vi "BioMap_BinaryFormat.vi"(11 "Binary file path":path) -> ()   [LabVIEW 2014]
uses:
  ControlDef/ProcessingMode.ctl
  Files/Signal_Segment.ctl
  Files/BinaryHeader_v31.ctl
  _BinaryFileViewer/BinaryRead_State.ctl
  _BinaryFileViewer/ReaderUpperLevelRefs.ctl
  _BinaryFileViewer/BinaryReader_Params.ctl
  preProc_State.ctl
  ControlDef/SampleRateSelector.ctl
  Files/BinaryHeader.ctl
  Apps/Apps_static/ScanParams_SingleLine.ctl
  Apps/ImagingMS/Imaging_Params.ctl
  ProcessMethods/SignalAverager/ProcessStates.ctl
  ControlDef/Signal.ctl
  ControlDef/LaserCtrl_Method.ctl
  ControlDef/States-AToF.ctl
  <instrlib>/ESP300/Public/Data/ESP300_State.ctl
  <instrlib>/ESP300/ESP300.lvlib
  <instrlib>/DG535/Command/DG535_States.ctl
  <instrlib>/DG535/SRS_DG535_Lib.lvlib
  Hardware/BNC(QuantumComposers)/BNC_States.ctl
  Hardware/FemtoLaser(Legacy)/Laser_Status.ctl
  Hardware/DAQmx(Legacy)/DAQmx_Status.ctl
  Files/WriterState.ctl
  Hardware/EPM2000(Legacy)/EPM2K_Status.ctl
  ControlDef/QueueRefs.ctl
  <vilib>/ptbypt/NI_PtbyPt.lvlib
  <instrlib>/GenericDAQ/VI/GenericDAQ_Signal.ctl
  <instrlib>/GenericDAQ/GenericDAQ.lvlib
  <instrlib>/GenericDAQ/VI/GenericDAQ_State.ctl
  <instrlib>/GenericDAQ/VI/GenericDAQ_Ctrl_Queue.ctl
panel:
  in  "Method":enum16{"Imaging (2D)", "Depth Profiling"}(ring)
  out "records/s":dbl format="%0.2f"
  out "CoreState":T1(ring)
  in  "Depth Overide":i32=-1
  in  "Rep.Rate (Hz)":dbl=10.0
  out "record count":i32
  in  "CheckHeader":bool
  in  "File Header":T2={"Start Position"=[], "StepWidth"=[0.05, 0.05], "Dimension"=[], "SpecLength"=10000}
  out "InvalidSpec":i32
  out "Percentage":dbl(slide) scale=0.0..100.0 scale format="%.1f"
  in  "Calibr.":dbl[](array[numeric])
  in  "ForceQuit":bool caption="Quit"
  in  "StartConv.":bool
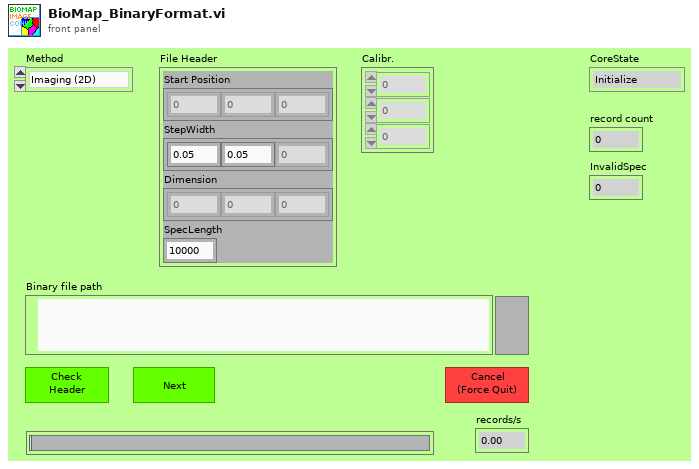
[diagram p1: front panel]
types:
  T1 = enum16{"Initialize", "Open", "Start", "Read", "Close", "Quit"}
  T2 = typedef "BinaryHeader_v31.ctl" = cluster{"Start Position":dbl[], "StepWidth":dbl[], "Dimension":i32[], "SpecLength":i32}
  T3 = typedef "BinaryReader_Params.ctl" = cluster{"FileVersion":string, "Start Position":dbl[], "StepWidth":dbl[], "Dimension":i32[], "TotalDepth":i32, "Spec#":u32, "FileSize":i64, "Calibr.":dbl[], "Position":dbl[], "Pressure":dbl, "Desp_LaserEnergy":dbl, "PI_LaserEnergy":dbl, "SpecLength":dbl, "Average#":i32, "SampleRate":dbl, "DAQ_Range":dbl, "Voltages Table":sgl[][], "ProcMode":T4, "Time Stamp":timestamp, "TrigDelay":dbl, "TickCount":dbl}
  T4 = typedef "ProcessingMode.ctl" = enum16{"None", "Drop by Threshold", "TDC Simulate", "SetFilter"}
  T5 = cluster{"PIEnergyCorrect":bool, "TBD":bool, "SpecLength":i32, "HeaderRefs":refnum<vi>, "Header":T3, "BioMAP file path":path, "InvalidSpec":refnum<vi>, "Calibr.Ref":refnum<vi>, "File Header":refnum<vi>, "QuitUserEvent":refnum<user-event>, "Proc/Signal_CoreQueue":refnum<queue>, "DynamicParams_Queue":refnum<queue>, "WriterQueue":refnum<queue>, "ProcessorHandle":refnum<vi>, "BufferRefs":refnum<queue>}
  T6 = typedef "preProc_State.ctl" = cluster{"State":enum16{"Initialize", "Open", "Start", "Read", "Close", "Quit"}, "Para.":variant}
  T7 = typedef "ReaderUpperLevelRefs.ctl" = cluster{"Percentage":refnum<vi>, "ForceQuit":refnum<vi>, "Header":refnum<vi>}
  T8 = typedef "Signal_Segment.ctl" = cluster{"SampleRate":dbl, "TrigDelay":dbl, "SpecLength":dbl, "DAQ_Range":dbl, "Average#":i32, "Position":dbl[], "Spectrum":sgl[], "Calibr.":dbl[], "Pressure":dbl, "Desp_LaserEnergy":dbl, "PI_LaserEnergy":dbl, "Voltages Table":sgl[][], "ProcMode":T4, "Threshold":dbl, "Comment":string, "TickCount":dbl, "Time Stamp":timestamp}
  T9 = typedef "BinaryRead_State.ctl" = cluster{"State":enum16{"Open", "GetHeader", "Index", "Read_i", "Read_all", "Close", "Quit"}, "Params":variant}
  T10 = cluster{"Image file path":path, "Binary file path":path}
  T11 = typedef "QueueRefs.ctl" = cluster{"LaserCtrlMethod":T12, "Apps":refnum<queue>, "MainDAQCoreQueue":refnum<queue>, "Micos":refnum<queue>, "ESP300":refnum<queue>, "SMC100":refnum<queue>, "SRS DG535":refnum<queue>, "BNC":refnum<queue>, "SDG_ii":refnum<queue>, "NI-USB_DAQmx":refnum<queue>, "ProcCore_CtrlQueue":refnum<queue>, "WriterCtrl":refnum<queue>, "WriterSIG":refnum<queue>, "Feedback":refnum<queue>, "EPM2000":refnum<queue>, "InfoRef":refnum<vi>, "AppsLock":T13, "ProcCore_SignalBuffer":refnum<queue>}
  T12 = typedef "LaserCtrl_Method.ctl" = enum16{"SRS_DG535", "BNC", "SDG_II", "GenericDAQ_Sim"}
  T13 = typedef "Semaphore RefNum" = refnum<k1>
  T14 = typedef "Signal.ctl" = cluster{"Command":T15, "Params":variant}
  T15 = typedef "ProcessStates.ctl" = enum16{"Initialize", "Normal", "Display", "Write2Buffer", "CalcMzArray", "StartSave", "StopSave", "ConfigChanged", "EndOfLine", "SetFilterParams", "SetGraphsEnable", "SetAcquisitionParams", "ChangeDisplayIncrement", "ChangeRepRate", "SetWriterRef", "Quit", "StartOfLine"}
  T16 = typedef "Imaging_Params.ctl" = cluster{"File Header":T17, "ScanSpeed":dbl, "HighSpeed":dbl, "SampleRate":T18, "Rep.Rate (Hz)":dbl, "TrigDelay":dbl, "mzCali":dbl[], "KeepStill(ms)":u32, "SaveRaw":bool, "MultiRec":bool}
  T17 = typedef "BinaryHeader.ctl" = cluster{"Start Position":dbl[], "StepWidth":dbl[], "Dimension":i32[], "SpecLength":i32}
  T18 = typedef "SampleRateSelector.ctl" = dbl
  T19 = typedef "ScanParams_SingleLine.ctl" = cluster{"Line Start":dbl[], "Line End":dbl[], "HighSpeed":dbl, "ScanSpeed":dbl, "KeepStill(ms)":u32, "SecendaryParams":variant}
  T20 = cluster{"queue out":refnum<queue>, "queue out":refnum<queue>}
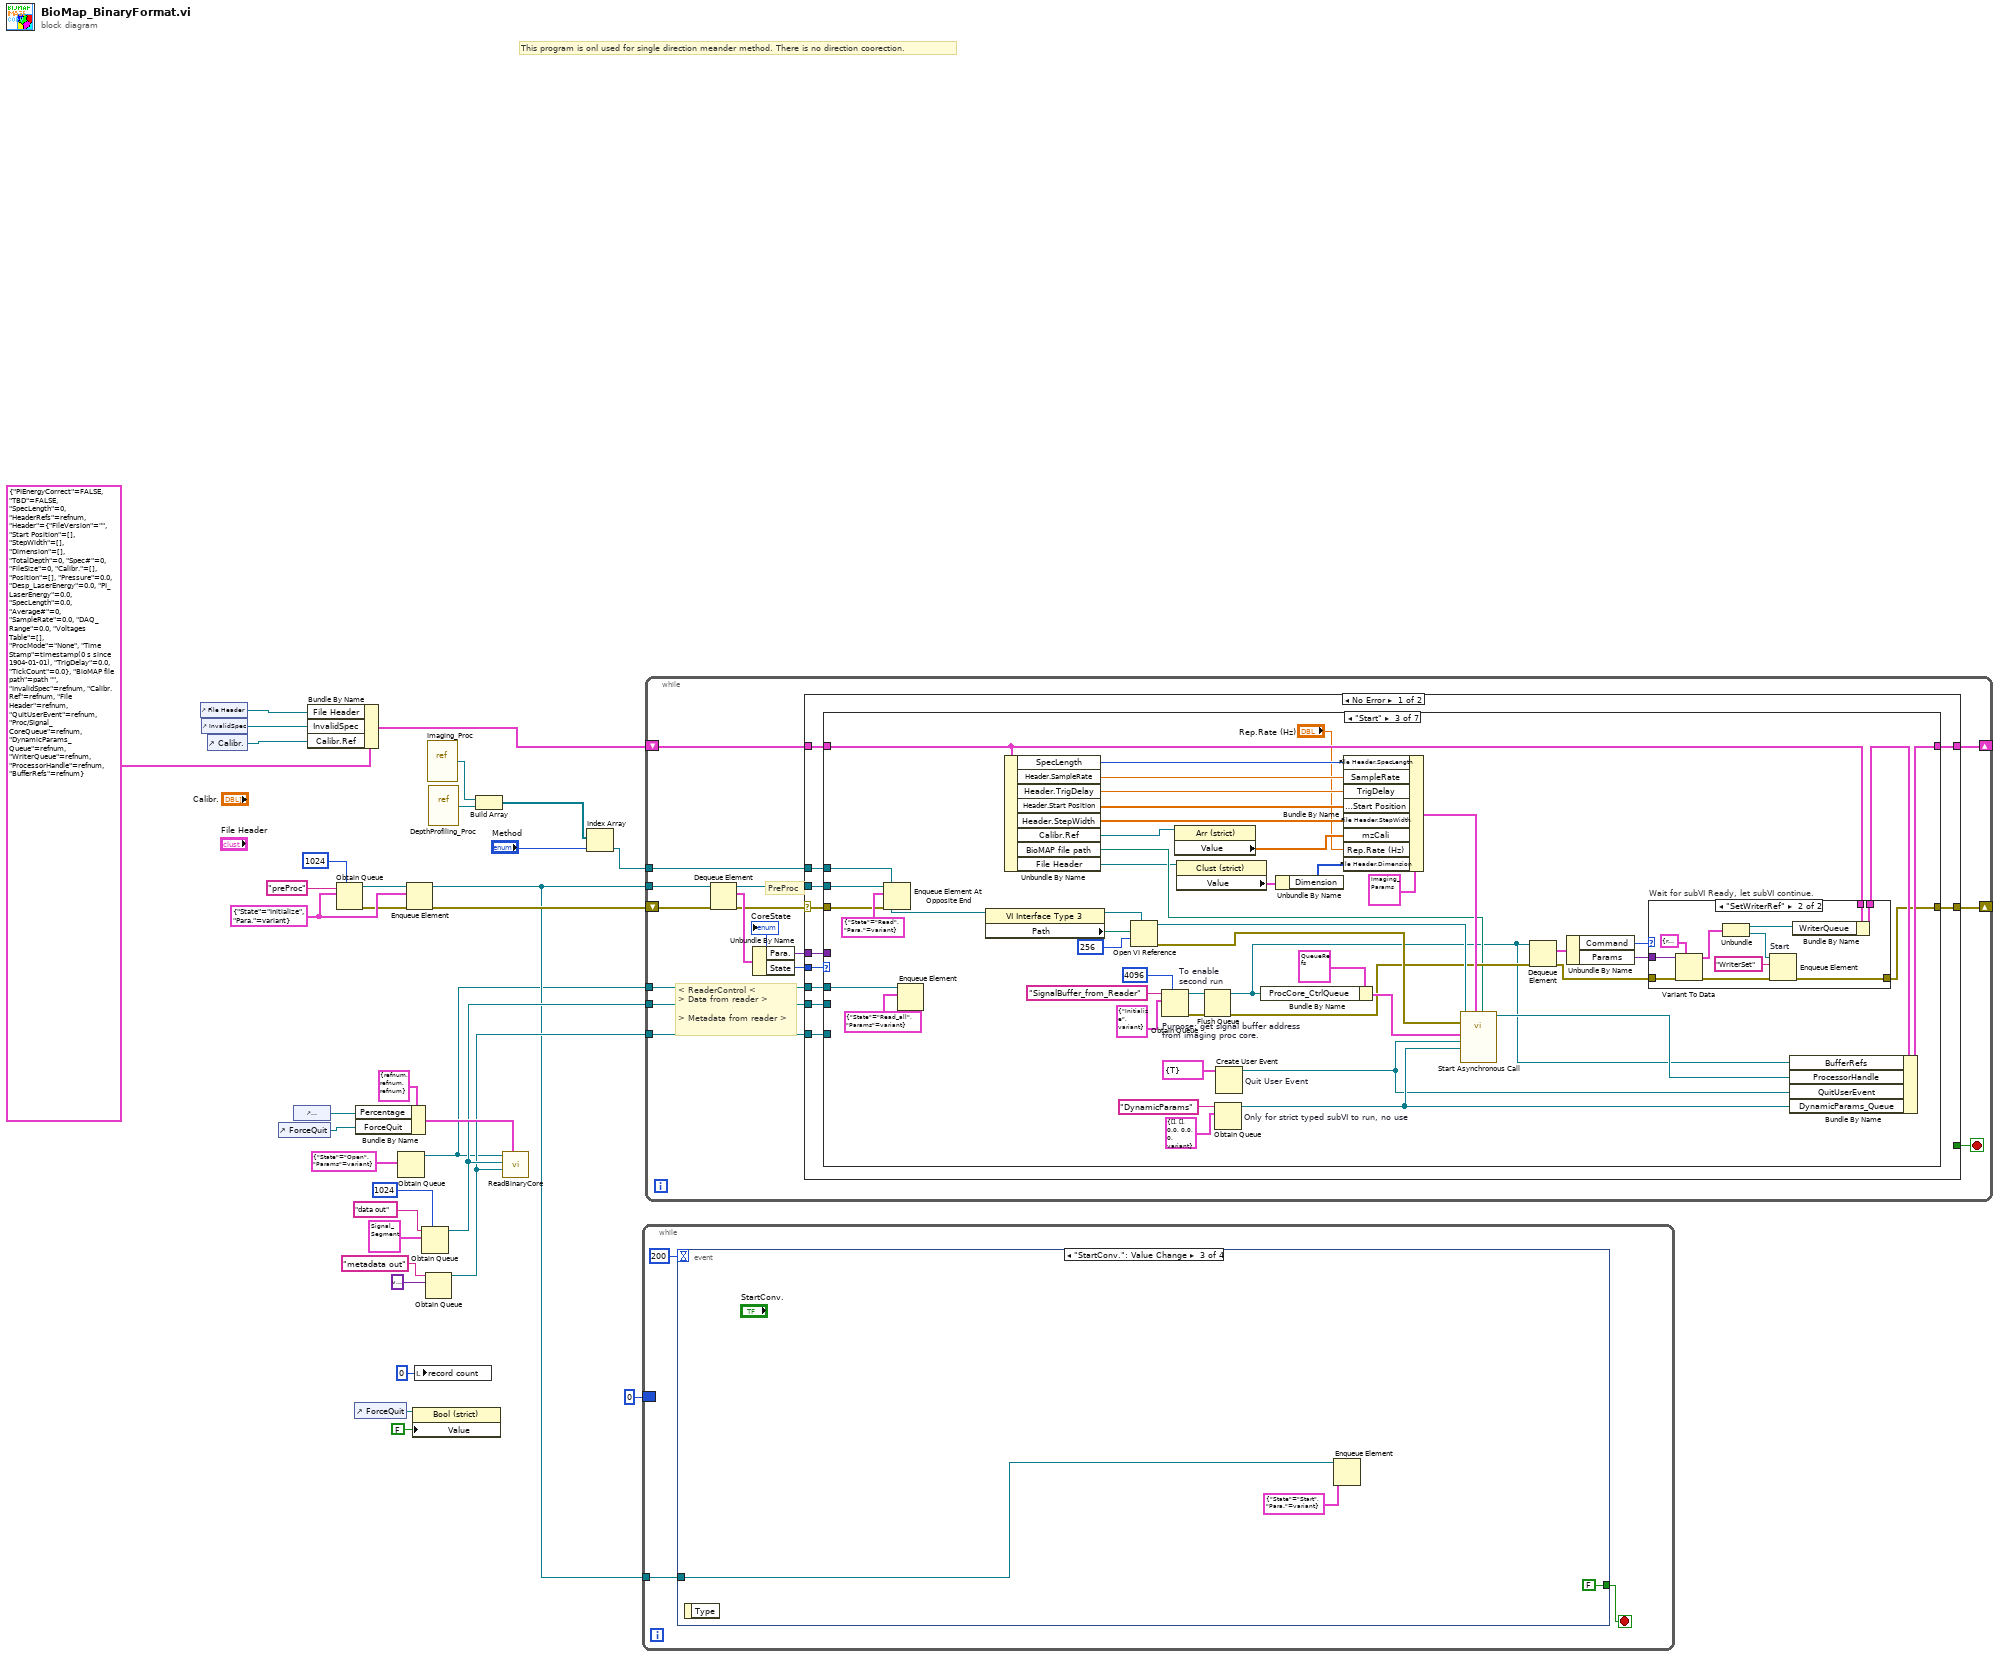
[diagram p0: block diagram]
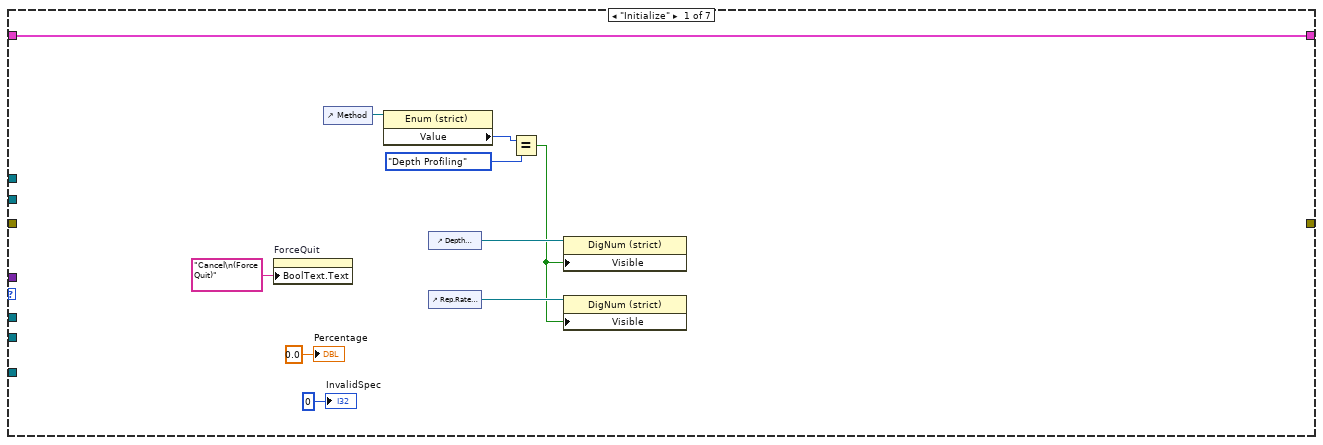
[diagram p2: hidden frame]
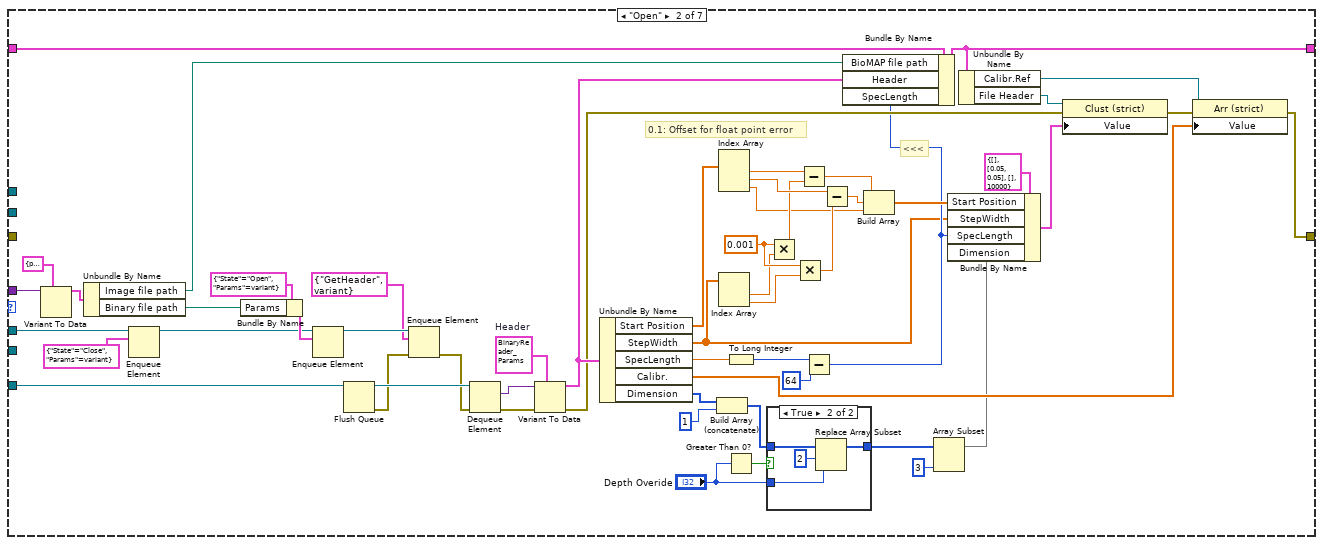
[diagram p3: hidden frame]
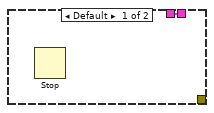
[diagram p5: hidden frame]
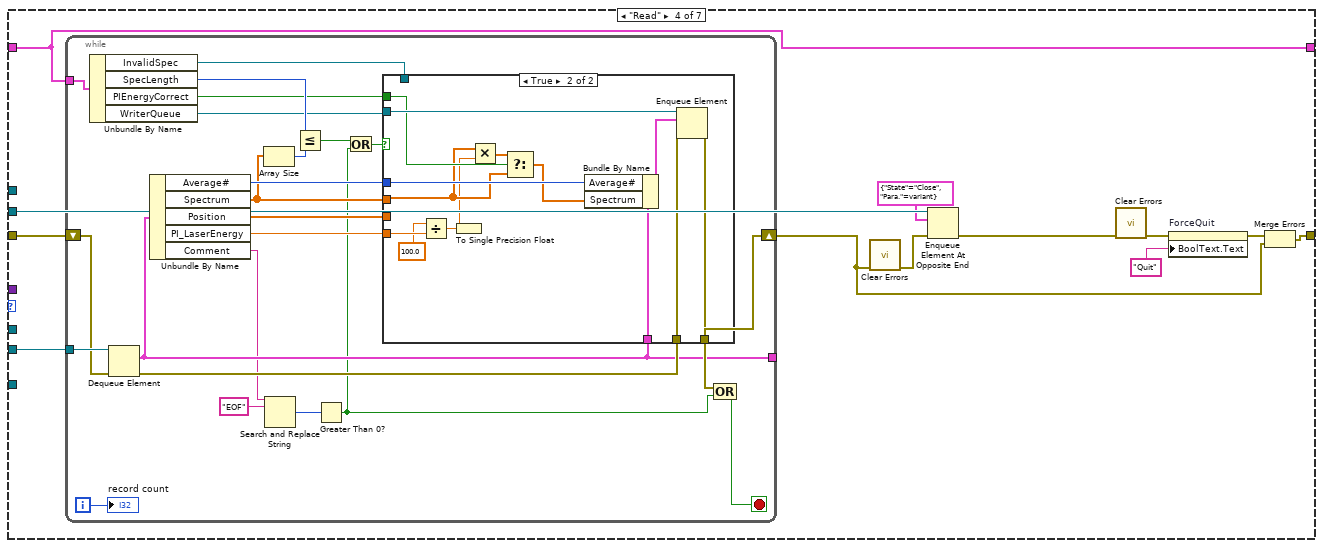
[diagram p6: hidden frame]
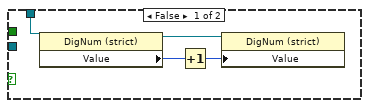
[diagram p7: hidden frame]
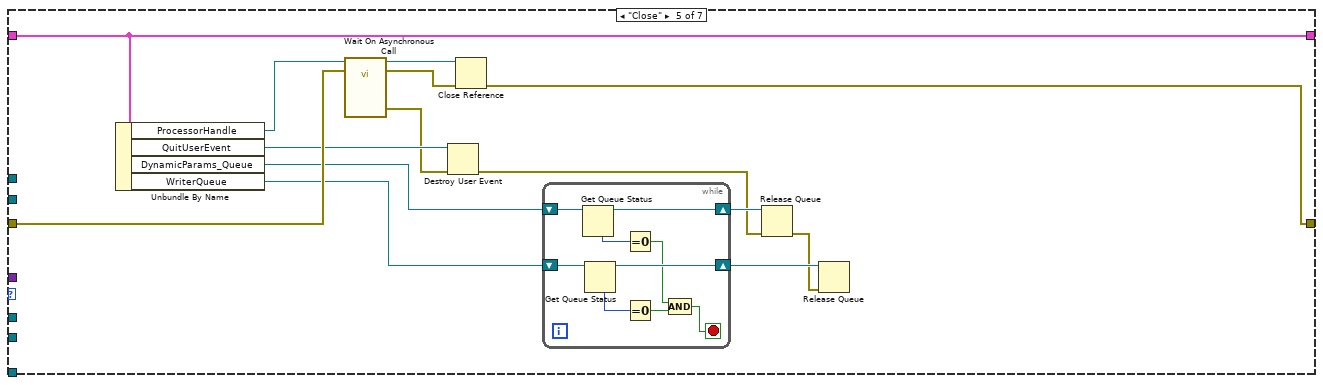
[diagram p8: hidden frame]
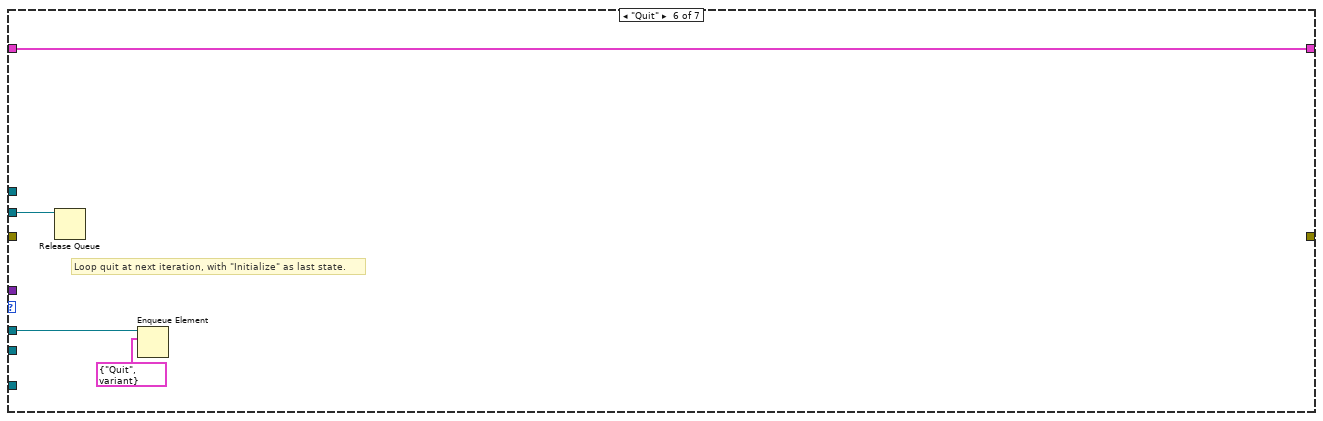
[diagram p9: hidden frame]
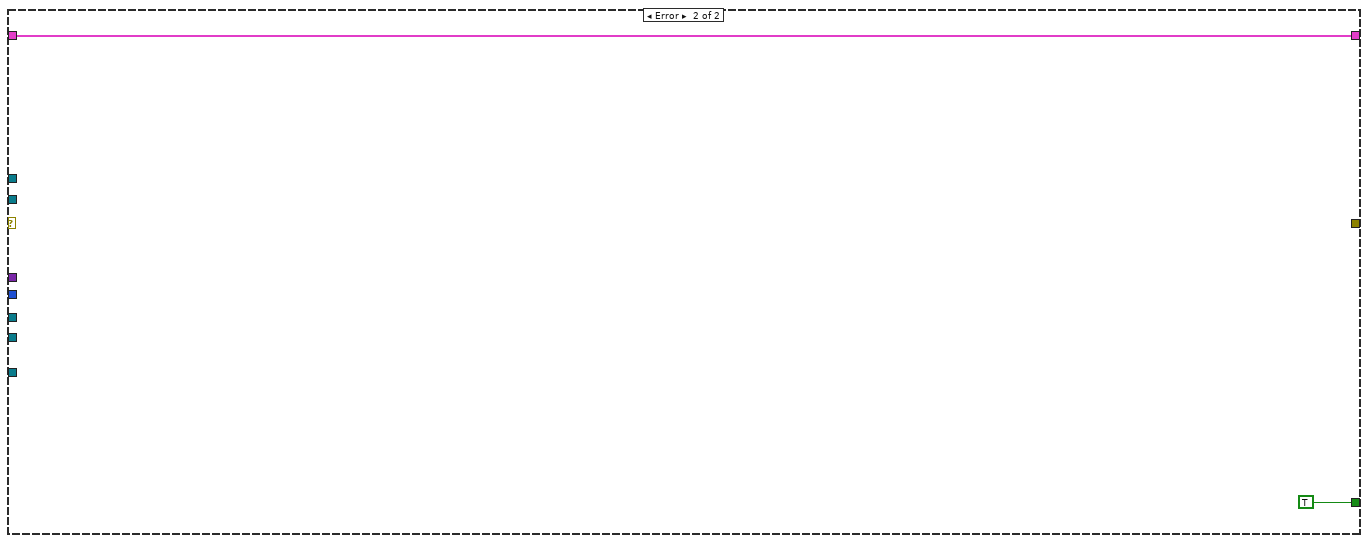
[diagram p11: hidden frame]
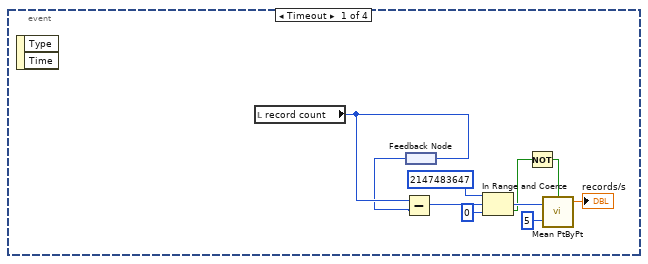
[diagram p12: hidden frame]
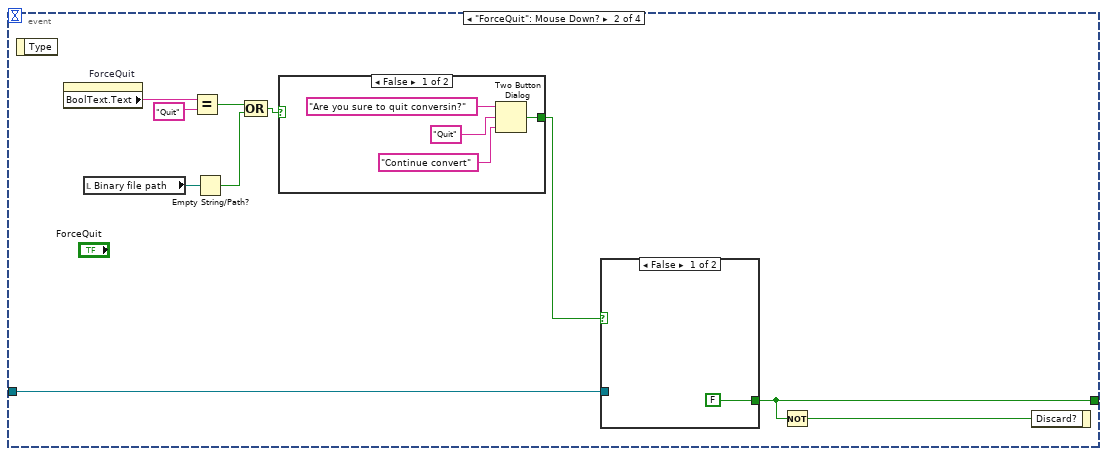
[diagram p13: hidden frame]
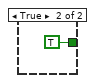
[diagram p14: hidden frame]
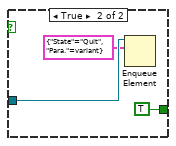
[diagram p15: hidden frame]
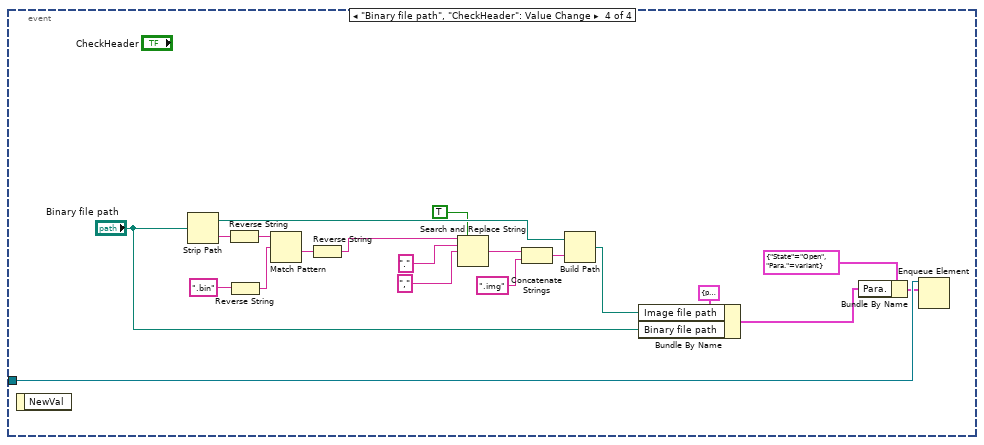
[diagram p16: hidden frame]
diagram:
  w26 = T6 {"State"=enum."Initialize", "Para."=variant}
  # "This program is onl used for single direction meander method. There is no direction coorection."
  n1 = control-ref of="File Header"() -> (w16:refnum<vi>)
  n2 = control-ref of="InvalidSpec"() -> (w19:refnum<vi>)
  n3 = control-ref of="Calibr."() -> (w20:refnum<vi>)
  n4 = control-ref of="ForceQuit"() -> (w14:refnum<vi>)
  n5 = control-ref of="Percentage"() -> (w32:refnum<vi>)
  n6 = Bundle By Name(cluster=T5 {"PIEnergyCorrect"=FALSE, "TBD"=FALSE, "SpecLength"=0, "HeaderRefs"=refnum, "Header"={"FileVersion"="", "Start Position"=[], "StepWidth"=[], "Dimension"=[], "TotalDepth"=0, "Spec#"=0, "FileSize"=0, "Calibr."=[], "Position"=[], "Pressure"=0.0, "Desp_LaserEnergy"=0.0, "PI_LaserEnergy"=0.0, "SpecLength"=0.0, "Average#"=0, "SampleRate"=0.0, "DAQ_Range"=0.0, "Voltages Table"=[], "ProcMode"=enum."None", "Time Stamp"=timestamp(0 s since 1904-01-01), "TrigDelay"=0.0, "TickCount"=0.0}, "BioMAP file path"=path "", "InvalidSpec"=refnum, "Calibr.Ref"=refnum, "File Header"=refnum, "QuitUserEvent"=refnum, "Proc/Signal_CoreQueue"=refnum, "DynamicParams_Queue"=refnum, "WriterQueue"=refnum, "ProcessorHandle"=refnum, "BufferRefs"=refnum}, "File Header"=w16, "InvalidSpec"=w19, "Calibr.Ref"=w20) -> (w17:T5)
  n7 = Obtain Queue(max queue size (-1, unlimited)=1024, name (unnamed)="preProc", element data type=w26) -> (queue out=w24:refnum<queue>, error out=w25:errorcluster)  [unwired: 2 in, 1 out]
  n8 = control-ref of="ForceQuit"() -> (w12:refnum<vi>)
  n9 = Bundle By Name(cluster=T7 {"Percentage"=refnum, "ForceQuit"=refnum, "Header"=refnum}, "Percentage"=w32, "ForceQuit"=w14) -> (w30:T7)
  n10 = Obtain Queue(element data type=T9 {"State"=enum."Open", "Params"=variant}) -> (queue out=w13:refnum<queue>)  [unwired: 4 in, 2 out]
  n11 = Enqueue Element(queue=w24, element=w26, error in (no error)=w25) -> (queue out=w15:refnum<queue>, error out=w23:errorcluster)  [unwired: 1 in, 1 out]
  n12 = property class="Bool (strict)"(reference=w12, "Value"=FALSE) -> ()  [unwired: 1 in, 2 out]
  n13 = local write "record count"(0 ("record count")) -> ()
  n14 = Obtain Queue(max queue size (-1, unlimited)=1024, name (unnamed)="data out", element data type=T8 {"SampleRate"=0.0, "TrigDelay"=0.0, "SpecLength"=0.0, "DAQ_Range"=0.0, "Average#"=0, "Position"=[], "Spectrum"=[], "Calibr."=[], "Pressure"=0.0, "Desp_LaserEnergy"=0.0, "PI_LaserEnergy"=0.0, "Voltages Table"=[], "ProcMode"=enum."None", "Threshold"=0.0, "Comment"="", "TickCount"=0.0, "Time Stamp"=timestamp(0 s since 1904-01-01)} ("Signal Segment")) -> (queue out=w29:refnum<queue>)  [unwired: 2 in, 2 out]
  n15 = Obtain Queue(name (unnamed)="metadata out", element data type=variant) -> (queue out=w21:refnum<queue>)  [unwired: 3 in, 2 out]
  n16 = vi-ref "Imaging_Proc.vi"() -> (w5:refnum<vi>)
  n17 = vi-ref "DepthProfiling_Proc.vi"() -> (w4:refnum<vi>)
  n18 = Build Array(w5, w4) -> (w2:refnum<vi>[])
  n19 = call "ReadBinaryCore.vi"("UpperLevelControlRefs."=w30, "metadata in"=w21, "data out in"=w29, "Control Queue in"=w13) -> ()  [unwired: 8 in]
  n20 = Index Array(array=w2, index="Method") -> (element=w3:refnum<vi>)
  n21 = while {
    tunnel: w15 -> [w36]
    border: 0 ("record count") -> [_]
    stop <- w37 stop-if-true
    n22 = event shown="[2] \"StartConv.\": Value Change" {
      selector: _ -> [_ _ _ _]
      dyn-events: _ -> [_ _ _ _]
      timeout: 200 -> [_ _ _ _]
      tunnel: [_ w57 FALSE _] -> w37
      tunnel: w36 -> [_ w48 w69 w81]
      event Timeout {
        n23 = event-data() -> ()  [unwired: 1 in, 2 out]
        n24 = local read "record count"() -> (w44:i32)
        n25 = feedback-in #1(w44) -> ()
        n26 = feedback #1() -> (w43:i32)
        n27 = Subtract(x=w44, y=w43) -> (x-y=w47:i32)
        n28 = In Range and Coerce(upper limit=2147483647, x=w47, lower limit=0) -> (coerced(x)=w42:i32, In Range?=w39:bool)
        n29 = Not(x=w39) -> (.not. x?=w38:bool)
        n30 = call <vilib>:"Mean PtByPt.vi"("x"=w42, "sample length"=5, "initialize"=w38) -> ("mean"=→"records/s":dbl)  [unwired: 1 in, 1 out]
      }
      event "ForceQuit": Mouse Down? {
        n31 = event-data() -> ()  [unwired: 1 in, 1 out]
        n32 = property on="ForceQuit" class="Bool (strict)"() -> ("BoolText.Text"=w53:string)  [unwired: 2 in, 2 out]
        n33 = local read "Binary file path"() -> (w52:path)
        n34 = Equal?(x=w53, y="Quit" ("Caption.Text")) -> (x = y?=w50:bool)
        n35 = Empty String/Path?(string/path=w52) -> (empty?=w49:bool)
        n36 = Compound Arithmetic op=OR(w50, w49) -> (w51:bool)
        n37 = case shown="False" w51 {
          tunnel: [w58 TRUE ("T button?")] -> w55
          frame False {
            n38 = Two Button Dialog(message="Are you sure to quit conversin?", 1:"Continue convert" ("F button name (\"Cancel\")"), 2:"Quit" ("T button name (\"OK\")")) -> (T button?=w58:bool)
          }
          frame True {
          }
        }
        n39 = case shown="False" w55 {
          tunnel: [FALSE TRUE] -> w57
          tunnel: w48 -> [_ w65]
          frame False {
          }
          frame True {
            n40 = Enqueue Element(queue=w65, element=T6 {"State"=enum."Quit", "Para."=variant}) -> ()  [unwired: 2 in, 3 out]
          }
        }
        n41 = Not(x=w57) -> (.not. x?=w56:bool)
        n42 = event-data("Discard?"=w56) -> ()  [unwired: 1 in, 1 out]
      }
      event "StartConv.": Value Change {
        n43 = event-data() -> ()  [unwired: 1 in, 1 out]
        n44 = Enqueue Element(queue=w69, element=T6 {"State"=enum."Start", "Para."=variant}) -> ()  [unwired: 2 in, 3 out]
      }
      event "Binary file path", "CheckHeader": Value Change {
        n45 = event-data() -> ()  [unwired: 1 in, 1 out]
        n46 = Strip Path(path="Binary file path") -> (stripped path=w82:path, name=w83:string)
        n47 = Reverse String(1:w83) -> (0:w89:string)
        n48 = Reverse String(1:".bin" ("regular expression")) -> (0:w84:string)
        n49 = Match Pattern(string=w89, regular expression=w84) -> (after substring=w86:string)  [unwired: 1 in, 3 out]
        n50 = Reverse String(1:w86) -> (0:w73:string)
        n51 = Search and Replace String(replace all?=TRUE ("replace all? (F)"), input string=w73, search string=".", replace string="," ("replace string (\"\")")) -> (result string=w74:string)  [unwired: 4 in, 3 out]
        n52 = Concatenate Strings(w74, ".img" ("string")) -> (w87:string)
        n53 = Build Path(base path=w82, name or relative path=w87) -> (appended path=w78:path)
        n54 = Bundle By Name(cluster=T10 {"Image file path"=path "", "Binary file path"=path ""} ("input cluster"), "Image file path"=w78, "Binary file path"="Binary file path") -> (w75:T10)
        n55 = Bundle By Name(cluster=T6 {"State"=enum."Open", "Para."=variant} ("element"), "Para."=w75) -> (w79:T6)
        n56 = Enqueue Element(queue=w81, element=w79) -> ()  [unwired: 2 in, 3 out]
      }
    }
  }
  n57 = while {
    tunnel: w29 -> [w104]
    tunnel: w15 -> [w102]
    shift-right: [w91] -> _
    shift-left: w23 -> [w103]
    tunnel: w13 -> [w98]
    shift-right: [w96] -> _
    shift-left: w17 -> [w95]
    tunnel: w21 -> [w94]
    tunnel: w3 -> [w90]
    stop <- w92 stop-if-true
    # "< ReaderControl <\n> Data from reader >\n\n> Metadata from reader >"
    # "PreProc"
    n58 = Dequeue Element(queue=w102, error in (no error)=w103) -> (queue out=w97:refnum<queue>, element=w101:T6, error out=w93:errorcluster)  [unwired: 1 in, 1 out]
    n59 = Unbundle By Name(w101) -> ("Para."=w99:variant, "State"=w100:T1)
    "CoreState" <- w100
    n60 = case shown="No Error" w93 {
      selector: w93 -> [w107 _]
      tunnel: w104 -> [w115 _]
      tunnel: w100 -> [w114 _]
      tunnel: w99 -> [w113 _]
      tunnel: w98 -> [w112 _]
      tunnel: w97 -> [w111 _]
      tunnel: [w110 w327] -> w96
      tunnel: w95 -> [w109 w327]
      tunnel: w94 -> [w108 _]
      tunnel: [_ TRUE] -> w92
      tunnel: [w106 _] -> w91
      tunnel: w90 -> [w105 _]
      frame No Error {
        n61 = case shown="\"Start\"" w114 {
          tunnel: w115 -> [_ _ _ w257 _ _ _]
          tunnel: w107 -> [_ _ w230 w256 w310 _ _]
          tunnel: w113 -> [_ w180 _ _ _ _ _]
          tunnel: w112 -> [_ w179 w204 _ _ w324 _]
          tunnel: w111 -> [_ _ w231 w255 _ w325 _]
          tunnel: [w122 w165 w212 w248 w312 w322 w326] -> w110
          tunnel: w109 -> [w122 w168 w209 w248 w312 w322 w326]
          tunnel: w108 -> [_ w175 _ _ _ _ _]
          tunnel: [_ w142 w199 w250 w307 _ _] -> w106
          tunnel: w105 -> [_ _ w192 _ _ _ _]
          frame "Initialize" {
            n62 = property on="ForceQuit" class="Bool (strict)"("BoolText.Text"="Cancel\n(Force Quit)" ("Caption.Text")) -> ()  [unwired: 2 in, 2 out]
            n63 = control-ref of="Method"() -> (w119:refnum<vi>)
            n64 = property class="Enum (strict)"(reference=w119) -> ("Value"=w118:enum16{"Imaging (2D)", "Depth Profiling"})  [unwired: 1 in, 2 out]
            n65 = control-ref of="Depth Overide"() -> (w121:refnum<vi>)
            n66 = control-ref of="Rep.Rate (Hz)"() -> (w120:refnum<vi>)
            n67 = Equal?(x=w118, y=enum16{"Imaging (2D)", "Depth Profiling"}."Depth Profiling") -> (x = y?=w116:bool)
            n68 = property class="DigNum (strict)"(reference=w121, "Visible"=w116) -> ()  [unwired: 1 in, 2 out]
            n69 = property class="DigNum (strict)"(reference=w120, "Visible"=w116) -> ()  [unwired: 1 in, 2 out]
            "Percentage" <- 0.0 ("Percentage")
            "InvalidSpec" <- 0 ("InvalidSpec")
          }
          frame "Open" {
            w161 = 0.001 ("x")
            w170 = T3 {"FileVersion"="", "Start Position"=[], "StepWidth"=[], "Dimension"=[], "TotalDepth"=0, "Spec#"=0, "FileSize"=0, "Calibr."=[], "Position"=[], "Pressure"=0.0, "Desp_LaserEnergy"=0.0, "PI_LaserEnergy"=0.0, "SpecLength"=0.0, "Average#"=0, "SampleRate"=0.0, "DAQ_Range"=0.0, "Voltages Table"=[], "ProcMode"=enum."None", "Time Stamp"=timestamp(0 s since 1904-01-01), "TrigDelay"=0.0, "TickCount"=0.0}  # Header
            # "<<<"
            # "0.1: Offset for float point error"
            n70 = Variant To Data(type=T10 {"Image file path"=path "", "Binary file path"=path ""} ("input cluster"), Variant=w180) -> (data=w139:T10)  [unwired: 1 in, 1 out]
            n71 = Unbundle By Name(w139) -> ("Image file path"=w137:path, "Binary file path"=w138:path)
            n72 = Enqueue Element(queue=w179, element=T9 {"State"=enum."Close", "Params"=variant}) -> (queue out=w167:refnum<queue>)  [unwired: 2 in, 2 out]
            n73 = Bundle By Name(cluster=T9 {"State"=enum."Open", "Params"=variant} ("element"), "Params"=w138) -> (w177:T9)
            n74 = Enqueue Element(queue=w167, element=w177) -> (queue out=w176:refnum<queue>)  [unwired: 2 in, 2 out]
            n75 = Flush Queue(queue=w175) -> (queue out=w174:refnum<queue>, error out=w173:errorcluster)  [unwired: 1 in, 1 out]
            n76 = Enqueue Element(queue=w176, element=T9 {"State"=enum."GetHeader", "Params"=variant}, error in (no error)=w173) -> (error out=w172:errorcluster)  [unwired: 1 in, 2 out]
            n77 = Dequeue Element(queue=w174, error in (no error)=w172) -> (element=w171:variant, error out=w169:errorcluster)  [unwired: 1 in, 2 out]
            n78 = Variant To Data(error in=w169, type=w170, Variant=w171) -> (data=w150:T3, error out=w141:errorcluster)
            n79 = Unbundle By Name(w150) -> ("Start Position"=w155:dbl[], "StepWidth"=w134:dbl[], "SpecLength"=w152:dbl, "Calibr."=w144:dbl[], "Dimension"=w133:i32[])
            n80 = Build Array (concatenate)(w133, 1) -> (w129:i32[])
            n81 = Index Array(array=w155) -> (element #1=w154:dbl, element #2=w162:dbl, element #3=w135:dbl)  [unwired: 3 in]
            n82 = Index Array(array=w134) -> (element #1=w160:dbl, element #2=w163:dbl)  [unwired: 2 in]
            n83 = To Long Integer(number=w152) -> (32bit integer=w151:i32)
            n84 = Greater Than 0?(x="Depth Overide") -> (x > 0?=w130:bool)
            n85 = case shown="True" w130 {
              tunnel: w129 -> [w181 w185]
              tunnel: [w181 w184] -> w132
              tunnel: "Depth Overide" -> [_ w182]
              frame False {
              }
              frame True {
                n86 = Replace Array Subset(array=w185, new element=w182, index=2) -> (w184:i32[])
              }
            }
            n87 = Multiply(x=w161, y=w160) -> (x*y=w158:dbl)
            n88 = Multiply(x=w161, y=w163) -> (x*y=w159:dbl)
            n89 = Subtract(x=w154, y=w158) -> (x-y=w156:dbl)
            n90 = Subtract(x=w151, y=64 ("x")) -> (x-y=w136:i32)
            n91 = Subtract(x=w162, y=w159) -> (x-y=w157:dbl)
            n92 = Bundle By Name(cluster=w168, "BioMAP file path"=w137, "Header"=w150, "SpecLength"=w136) -> (w165:T5)
            n93 = Build Array(w156, w157, w135) -> (w149:dbl[])
            n94 = Array Subset(array=w132, length=3) -> (w127:i32[])  [unwired: 1 in]
            n95 = Bundle By Name(cluster=T2 {"Start Position"=[], "StepWidth"=[0.05, 0.05], "Dimension"=[], "SpecLength"=10000} ("File Header"), "Start Position"=w149, "StepWidth"=w134, "SpecLength"=w136, "Dimension"=w127) -> (w148:T2)
            n96 = Unbundle By Name(w165) -> ("Calibr.Ref"=w145:refnum<vi>, "File Header"=w164:refnum<vi>)
            n97 = property class="Clust (strict)"(reference=w164, error in=w141, "Value"=w148) -> (error out=w146:errorcluster)  [unwired: 1 out]
            n98 = property class="Arr (strict)"(reference=w145, error in=w146, "Value"=w144) -> (error out=w142:errorcluster)  [unwired: 1 out]
          }
          frame "Start" {
            n99 = Enqueue Element At Opposite End(queue=w231, element=T6 {"State"=enum."Read", "Para."=variant}, error in (no error)=w230) -> ()  [unwired: 1 in, 3 out]
            n100 = Enqueue Element(queue=w204, element=T9 {"State"=enum."Read_all", "Params"=variant}) -> ()  [unwired: 2 in, 3 out]
            n101 = property class="VI Interface Type 3"(reference=w192) -> (reference out=w191:refnum<vi>, "Path"=w202:path)  [unwired: 1 in, 1 out]
            n102 = Unbundle By Name(w209) -> ("SpecLength"=w217:i32, "Header.SampleRate"=w218:dbl, "Header.TrigDelay"=w219:dbl, "Header.Start Position"=w221:dbl[], "Header.StepWidth"=w220:dbl[], "Calibr.Ref"=w216:refnum<vi>, "BioMAP file path"=w190:path, "File Header"=w189:refnum<vi>)
            n103 = Open VI Reference(type specifier VI Refnum (for type only)=w191, vi path=w202, options=256) -> (vi reference=w201:refnum<vi>, error out=w200:errorcluster)  [unwired: 3 in]
            n104 = Obtain Queue "Purpose: get signal buffer address \nfrom imaging proc core."(max queue size (-1, unlimited)=4096, name (unnamed)="SignalBuffer_from_Reader", element data type=T14 {"Command"=enum."Initialize", "Params"=variant} ("m/z signal")) -> (queue out=w214:refnum<queue>, error out=w195:errorcluster)  [unwired: 2 in, 1 out]
            n105 = property class="Arr (strict)"(reference=w216) -> ("Value"=w215:dbl[])  [unwired: 1 in, 2 out]
            n106 = property on="Property Node" class="Clust (strict)"(reference=w189) -> ("Value"=w188:T2)  [unwired: 1 in, 2 out]
            n107 = Flush Queue "To enable\nsecond run"(queue=w214, error in (no error)=w195) -> (queue out=w186:refnum<queue>, error out=w194:errorcluster)  [unwired: 1 out]
            n108 = Obtain Queue "Only for strict typed subVI to run, no use"(name (unnamed)="DynamicParams", element data type=T19 {"Line Start"=[], "Line End"=[], "HighSpeed"=0.0, "ScanSpeed"=0.0, "KeepStill(ms)"=0, "SecendaryParams"=variant(dbl[] [])}) -> (queue out=w207:refnum<queue>)  [unwired: 3 in, 2 out]
            n109 = Create User Event "Quit User Event"(user event datatype=cluster{"Quit":bool} {"Quit"=TRUE} ("Quit")) -> (user event=w205:refnum<user-event>)  [unwired: 1 in, 1 out]
            n110 = Bundle By Name(cluster=T11 {"LaserCtrlMethod"=enum."SRS_DG535", "Apps"=refnum, "MainDAQCoreQueue"=refnum, "Micos"=refnum, "ESP300"=refnum, "SMC100"=refnum, "SRS DG535"=refnum, "BNC"=refnum, "SDG_ii"=refnum, "NI-USB_DAQmx"=refnum, "ProcCore_CtrlQueue"=refnum, "WriterCtrl"=refnum, "WriterSIG"=refnum, "Feedback"=refnum, "EPM2000"=refnum, "InfoRef"=refnum, "AppsLock"=refnum, "ProcCore_SignalBuffer"=refnum} ("QueuesRef"), "ProcCore_CtrlQueue"=w186) -> (w198:T11)
            n111 = Unbundle By Name(w188) -> ("Dimension"=w187:i32[])
            n112 = Bundle By Name(cluster=T16 {"File Header"={"Start Position"=[], "StepWidth"=[], "Dimension"=[], "SpecLength"=0}, "ScanSpeed"=0.0, "HighSpeed"=0.0, "SampleRate"=0.0, "Rep.Rate (Hz)"=0.0, "TrigDelay"=0.0, "mzCali"=[], "KeepStill(ms)"=0, "SaveRaw"=FALSE, "MultiRec"=FALSE} ("BeamProfiling_Params"), "File Header.SpecLength"=w217, "SampleRate"=w218, "TrigDelay"=w219, "File Header.Start Position"=w221, "File Header.StepWidth"=w220, "mzCali"=w215, "Rep.Rate (Hz)"="Rep.Rate (Hz)", "File Header.Dimension"=w187) -> (w229:T16)
            n113 = call-by-ref "Start Asynchronous Call"(reference=w201, error in=w200, "DP_filepath"=w190, "Params."=w229, "Dynamic Params In"=w207, "Quit_UserEvent"=w205, "ControlQueueRef"=w198) -> (reference out=w196:refnum<vi>)  [unwired: 5 in, 3 out]
            n114 = Dequeue Element(queue=w186, error in (no error)=w194) -> (element=w213:T14, error out=w193:errorcluster)  [unwired: 1 in, 2 out]
            n115 = Unbundle By Name(w213) -> ("Command"=w211:T15, "Params"=w210:variant)
            n116 = case "Wait for subVI Ready, let subVI continue." shown="\"SetWriterRef\"" w211 {
              tunnel: w209 -> [w234 w245]
              tunnel: w210 -> [_ w244]
              tunnel: [w234 w243] -> w208
              tunnel: [_ w237] -> w199
              tunnel: w193 -> [_ w235]
              frame Default {
                n117 = Stop() -> ()  [unwired: 1 in]
              }
              frame "SetWriterRef" {
                n118 = Variant To Data(error in=w235, type=T20 {"queue out"=refnum, "queue out"=refnum} ("cluster"), Variant=w244) -> (data=w241:T20, error out=w238:errorcluster)
                n119 = Unbundle(w241) -> ("queue out"=w240:refnum<queue>, "queue out"=w239:refnum<queue>)
                n120 = Enqueue Element "Start"(queue=w239, element="WriterSet", error in (no error)=w238) -> (error out=w237:errorcluster)  [unwired: 1 in, 2 out]
                n121 = Bundle By Name(cluster=w245, "WriterQueue"=w240) -> (w243:T5)
              }
            }
            n122 = Bundle By Name(cluster=w208, "BufferRefs"=w186, "ProcessorHandle"=w196, "QuitUserEvent"=w205, "DynamicParams_Queue"=w207) -> (w212:T5)
          }
          frame "Read" {
            n123 = while {
              tunnel: w257 -> [w280]
              shift-right: [w271] -> w249
              shift-left: w256 -> [w276]
              tunnel: w248 -> [w270]
              tunnel: [w263] -> _
              i -> [w264]
              stop <- w272 stop-if-true
              n124 = Unbundle By Name(w270) -> ("InvalidSpec"=w267:refnum<vi>, "SpecLength"=w269:i32, "PIEnergyCorrect"=w268:bool, "WriterQueue"=w266:refnum<queue>)
              n125 = Dequeue Element(queue=w280, error in (no error)=w276) -> (element=w263:T8, error out=w277:errorcluster)  [unwired: 1 in, 2 out]
              n126 = Unbundle By Name(w263) -> ("Average#"=w279:i32, "Spectrum"=w278:sgl[], "Position"=w265:dbl[], "PI_LaserEnergy"=w273:dbl, "Comment"=w262:string)
              n127 = Array Size(array=w278) -> (size(s)=w275:i32)
              n128 = Search and Replace String(input string=w262, search string="EOF" ("y")) -> (number of replacements=w260:i32)  [unwired: 6 in, 3 out]
              n129 = Less Or Equal?(x=w269, y=w275) -> (x <= y?=w274:bool)
              n130 = Greater Than 0?(x=w260) -> (x > 0?=w258:bool)
              n131 = Or(x=w274, y=w258) -> (x .or. y?=w259:bool)
              n132 = case shown="True" w259 {
                tunnel: w266 -> [_ w298]
                tunnel: w279 -> [_ w297]
                tunnel: w278 -> [_ w292]
                tunnel: w277 -> [_ w296]
                tunnel: w273 -> [_ w290]
                tunnel: w268 -> [_ w294]
                tunnel: [_ w288] -> w271
                tunnel: w267 -> [w284 _]
                tunnel: w263 -> [_ w286]
                tunnel: w265 -> [_ _]
                frame False {
                  n133 = property class="DigNum (strict)"(reference=w284) -> (reference out=w283:refnum<vi>, "Value"=w282:i32)  [unwired: 1 in, 1 out]
                  n134 = Increment(x=w282) -> (x+1=w281:i32)
                  n135 = property class="DigNum (strict)"(reference=w283, "Value"=w281) -> ()  [unwired: 1 in, 2 out]
                }
                frame True {
                  n136 = Divide(x=100.0, y=w290) -> (x/y=w291:dbl)
                  n137 = To Single Precision Float(number=w291) -> (single precision float=w287:sgl)
                  n138 = Multiply(x=w292, y=w287) -> (x*y=w293:sgl[])
                  n139 = Select(t=w293, s=w294, f=w292) -> (s? t:f=w295:sgl[])
                  n140 = Bundle By Name(cluster=w286, "Average#"=w297, "Spectrum"=w295) -> (w285:T8)
                  n141 = Enqueue Element(queue=w298, element=w285, error in (no error)=w296) -> (error out=w288:errorcluster)  [unwired: 1 in, 2 out]
                }
              }
              n142 = Compound Arithmetic op=OR(w271, w258) -> (w272:bool)
              "record count" <- w264
            }
            n143 = call <vilib>:"Clear Errors.vi"("error in (no error)"=w249) -> ("error out"=w247:errorcluster)  [unwired: 5 in, 1 out]
            n144 = Enqueue Element At Opposite End(queue=w255, element=T6 {"State"=enum."Close", "Para."=variant}, error in (no error)=w247) -> (error out=w246:errorcluster)  [unwired: 1 in, 2 out]
            n145 = call <vilib>:"Clear Errors.vi"("error in (no error)"=w246) -> ("error out"=w252:errorcluster)  [unwired: 5 in, 1 out]
            n146 = property on="ForceQuit" class="Bool (strict)"(error in=w252, "BoolText.Text"="Quit" ("Caption.Text")) -> (error out=w251:errorcluster)  [unwired: 1 in, 1 out]
            n147 = Merge Errors(w251, w249) -> (w250:errorcluster)
          }
          frame "Close" {
            n148 = Unbundle By Name(w312) -> ("ProcessorHandle"=w311:refnum<vi>, "QuitUserEvent"=w306:refnum<user-event>, "DynamicParams_Queue"=w305:refnum<queue>, "WriterQueue"=w303:refnum<queue>)
            n149 = call-by-ref "Wait On Asynchronous Call"(reference=w311, error in=w310) -> (reference out=w309:refnum<vi>, error out=w308:errorcluster, 0:"error out"=w304:errorcluster)  [unwired: 10 in, 1 out]
            n150 = Destroy User Event(user event=w306, error in=w304) -> (error out=w299:errorcluster)
            n151 = Close Reference(reference=w309, error in (no error)=w308) -> (error out=w307:errorcluster)
            n152 = while {
              shift-right: [w319] -> w302
              shift-left: w305 -> [w321]
              shift-right: [w318] -> w301
              shift-left: w303 -> [w320]
              stop <- w313 stop-if-true
              n153 = Get Queue Status(queue=w321) -> (queue out=w319:refnum<queue>, # elements in queue=w316:i32)  [unwired: 2 in, 6 out]
              n154 = Get Queue Status(queue=w320) -> (queue out=w318:refnum<queue>, # elements in queue=w317:i32)  [unwired: 2 in, 6 out]
              n155 = Equal To 0?(x=w316) -> (x = 0?=w314:bool)
              n156 = Equal To 0?(x=w317) -> (x = 0?=w315:bool)
              n157 = Compound Arithmetic op=AND(w314, w315) -> (w313:bool)
            }
            n158 = Release Queue(queue=w302, error in (no error)=w299) -> (error out=w300:errorcluster)  [unwired: 1 in, 2 out]
            n159 = Release Queue(queue=w301, error in (no error)=w300) -> ()  [unwired: 1 in, 3 out]
          }
          frame "Quit" {
            # "Loop quit at next iteration, with \"Initialize\" as last state."
            n160 = Release Queue(queue=w325) -> ()  [unwired: 2 in, 3 out]
            n161 = Enqueue Element(queue=w324, element=T9 {"State"=enum."Quit", "Params"=variant}) -> ()  [unwired: 2 in, 3 out]
          }
          frame Default {
          }
        }
      }
      frame Error {
      }
    }
  }
